vi "Line.vi"() -> ()   [LabVIEW 2021]
panel:
  in  "Checkbox":bool
  in  "Title":string
  in  "Comment":string
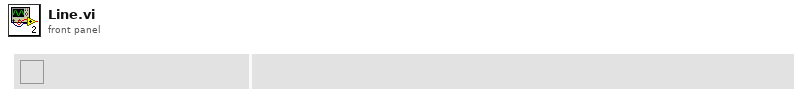
[diagram p1: front panel]
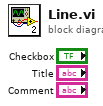
[diagram p0: block diagram]
diagram:
